vi "TellComponent.vi"(9 "ActorAlias":string, 10 "Message":refnum<class "Message.lvclass">, 11 "Actor":refnum<class "Actor.lvclass">) -> (3 "Actor":refnum<class "Actor.lvclass">)   [LabVIEW 2020, in "jettl.lvlib"]
uses:
  jettl.lvlib
  Actor/Actor.lvclass
  Message/Message.lvclass
  TellOrigin.ctl
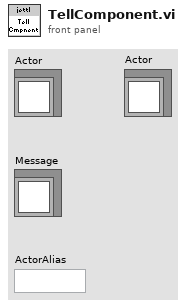
[diagram p1: front panel]
types:
  T1 = typedef "jettl.lvlib/TellOrigin.ctl" = enum16{"Self", "Mediator", "Component"}
  T2 = typedef "jettl.lvlib/Actor.ctl" = cluster{"Messages":T3, "ActorAlias":string, "ActorType":T6, "Transport":refnum<user-event>, "VIRef":refnum<vi>}
  T3 = typedef "jettl.lvlib/Messages.ctl" = cluster{"Listen":T4, "TellSelf":T4, "TellMediator":T4, "TellComponentMap":T5}
  T4 = typedef "jettl.lvlib/MessageSet.ctl" = set{refnum<class "Message.lvclass">}
  T5 = typedef "jettl.lvlib/TellComponentMap.ctl" = map{string, T4}
  T6 = typedef "jettl.lvlib/ActorType.ctl" = enum16{"Mediator", "Component"}
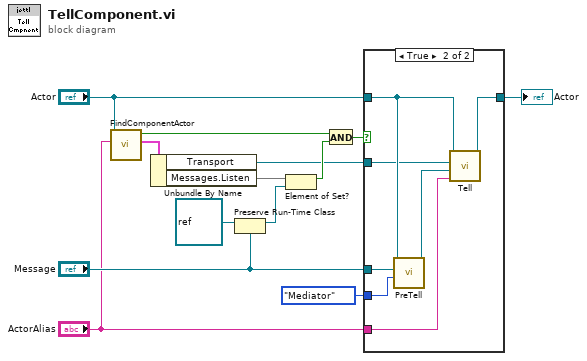
[diagram p0: block diagram]
diagram:
  n1 = call "FindComponentActor.vi"("ActorAlias"="ActorAlias", "Actor"="Actor") -> ("ComponentActor"=w5:T2, "Found"=w4:bool)  [unwired: 8 in]
  n2 = Unbundle By Name(w5) -> ("Transport"=w1:refnum<user-event>, "Messages.Listen"=w6:T4)
  n3 = Preserve Run-Time Class(object in=refnum<class> refnum, 2:"Message") -> (object out=w8:refnum<class "Message.lvclass">)  [unwired: 1 in, 1 out]
  n4 = Element of Set?(10:w8, 11:w6) -> (3:w12:bool)
  n5 = And(x=w4, y=w12) -> (x .and. y?=w11:bool)
  n6 = case shown="True" w11 {
    tunnel: "Actor" -> [w14 w17]
    tunnel: [w14 w21] -> w13
    tunnel: "ActorAlias" -> [_ w20]
    tunnel: "Message" -> [_ w19]
    tunnel: TellOrigin."Mediator" ("TellOrigin") -> [_ w18]
    tunnel: w1 -> [_ w15]
    frame False {
    }
    frame True {
      n7 = call "PreTell.vi"("TellOrigin"=w18, "Message"=w19, "Actor"=w17) -> ("Message"=w16:refnum<class "Message.lvclass">)  [unwired: 8 in]
      n8 = call "Tell.vi"("ActorAlias"=w20, "Message"=w16, "Transport"=w15, "Actor"=w17) -> ("Actor"=w21:refnum<class "Actor.lvclass">)  [unwired: 7 in]
    }
  }
  "Actor" <- w13
